vi "getPositionAllAxis.vi"(0 "connection ID":refnum<k5>, 5 "error":errorcluster) -> (14 "connection ID out":refnum<k5>, 15 "pos_nm_x":dbl, 16 "pos_nm_y":dbl, 17 "pos_nm_z":dbl, 19 "error out":errorcluster)   [LabVIEW 2016, in "amc_api.lvlib"]
doc: "This function returns the position of all three axes in nm\n If there is no positioner on one axis or the sensor is disabled, it returns -2147483648 nm instead"
uses:
  amc_api.lvlib
panel:
  out "jsonRespIn":string
  out "JSON-response":string="{\"jsonrpc\":\"2.0\",\"method\":\"\",\"params\":[5,1.245,true,\"name\"],\"id\":\"1\"}"
  out "JSON request":string
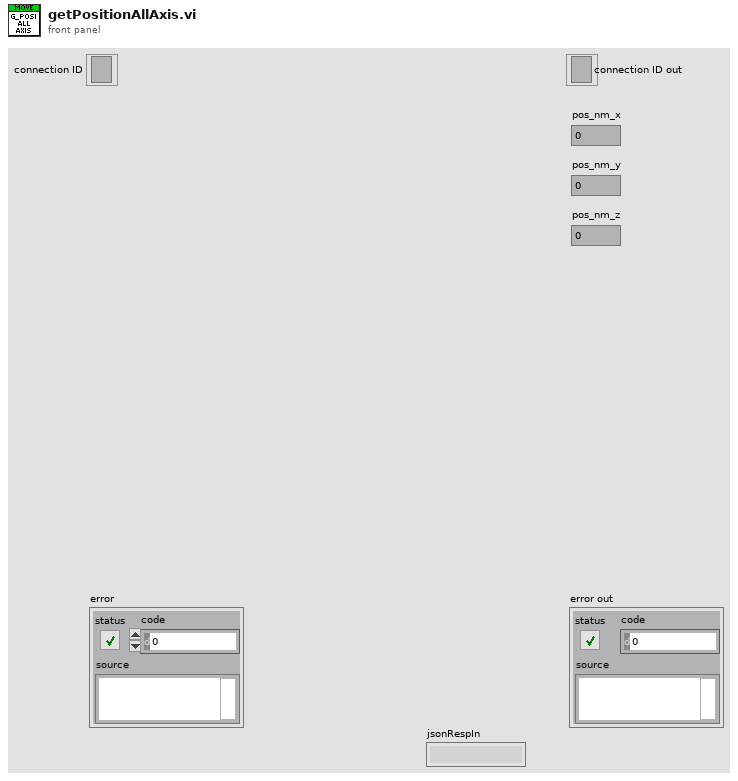
[diagram p1: front panel]
types:
  T1 = cluster{"jsonrpc":string, "method":string, "params":string[], "id":string, "api":i32, "pid":string}
  T2 = enum16{"Standard", "Buffered", "CRLF", "Immediate"}
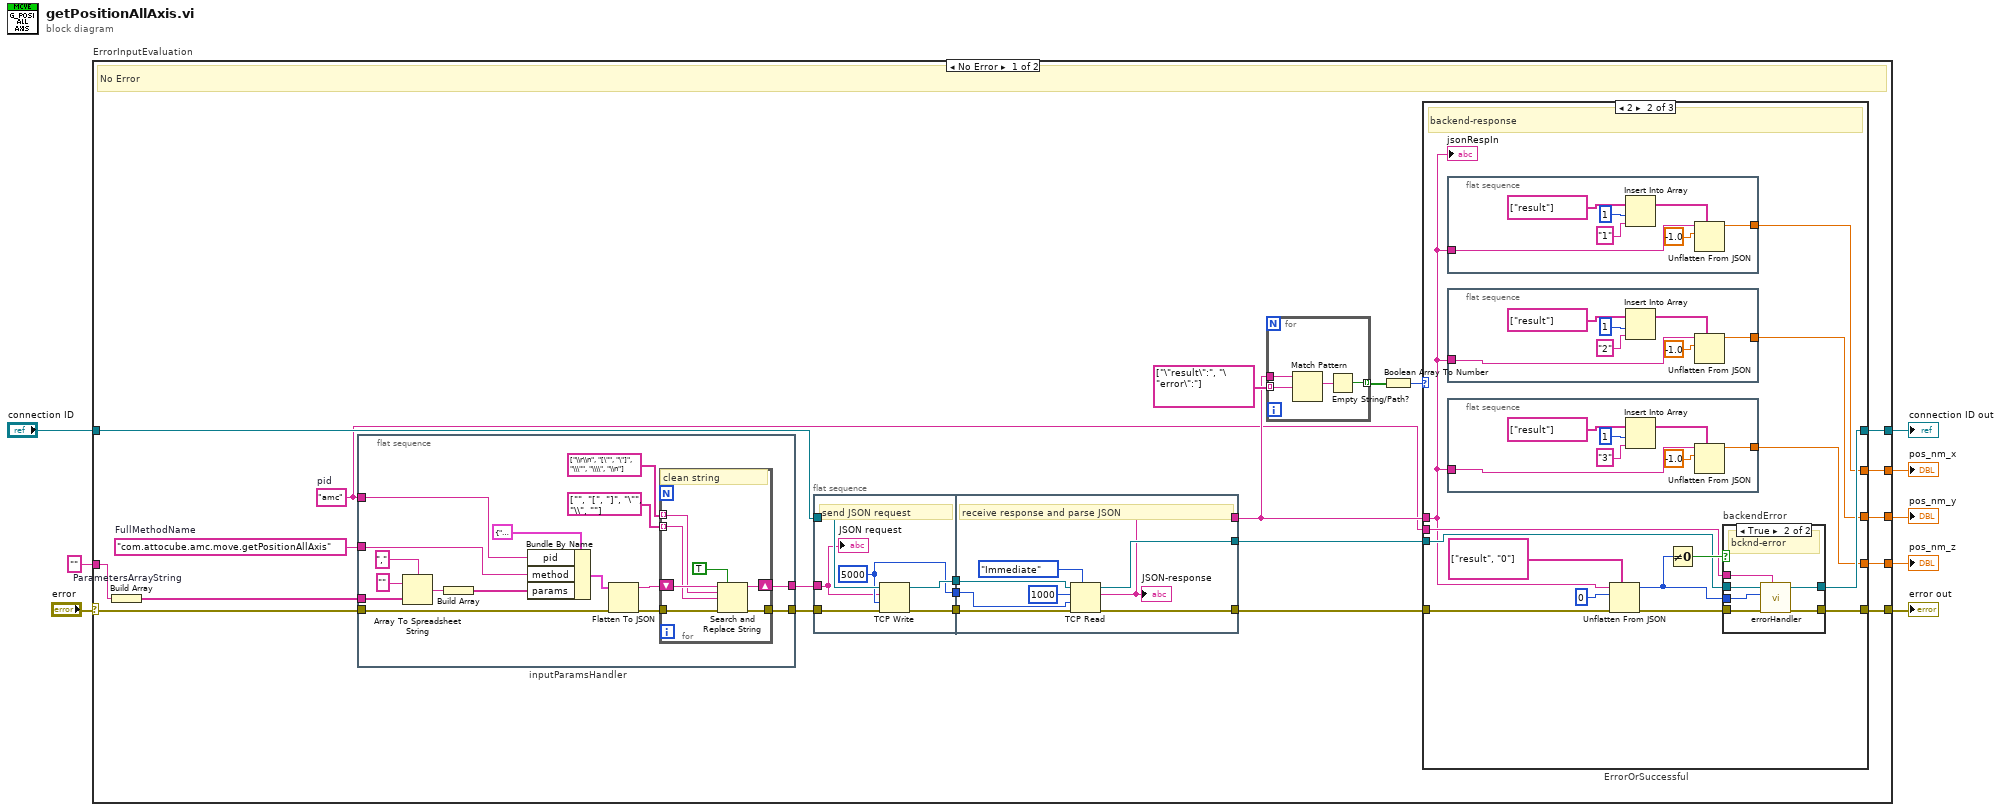
[diagram p0: block diagram]
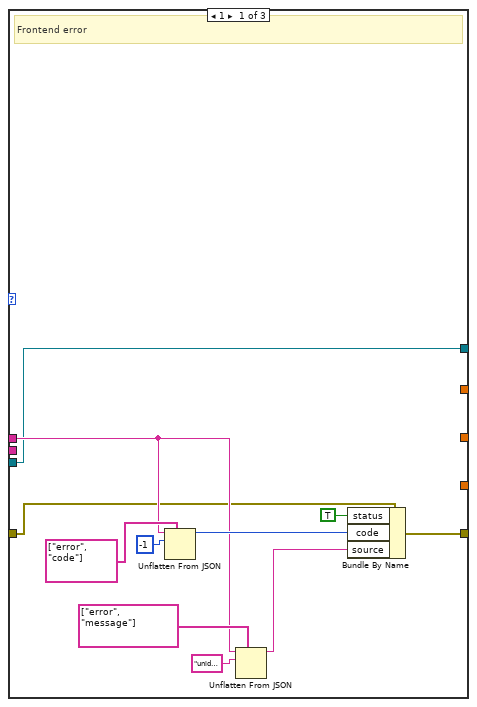
[diagram p2: hidden frame]
diagram:
  n1 = case "ErrorInputEvaluation" shown="No Error" "error" {
    selector: "error" -> [w23 w128]
    tunnel: "connection ID" -> [w27 w129]
    tunnel: [w14 w128] -> w7
    tunnel: [w15 w129] -> w6
    tunnel: "" -> [w12 _]
    tunnel: [w11 _] -> w3
    tunnel: [w10 _] -> w2
    tunnel: [w9 _] -> w1
    frame No Error {
      w13 = "amc"  # pid
      w24 = "com.attocube.amc.move.getPositionAllAxis"  # FullMethodName
      # "No Error"
      n2 = Build Array "ParametersArrayString"(w12) -> (w22:string[])
      n3 = flat-sequence "inputParamsHandler" {
        tunnel: [w92] -> w21
        tunnel: w22 -> [w98]
        tunnel: w23 -> [w97]
        tunnel: [w94] -> w20
        tunnel: w24 -> [w88]
        tunnel: w13 -> [w87]
        frame #0 {
          n4 = Array To Spreadsheet String(delimiter (Tab)=",", array=w98, 3:"" ("format string")) -> (spreadsheet string=w100:string)
          n5 = Build Array "Build Array"(w100) -> (w89:string[])
          n6 = Bundle By Name(cluster=T1 {"jsonrpc"="2.0", "method"="com.attocube.amc.res.setRESReadOutFreq", "params"=[], "id"="1", "api"=2, "pid"=""} ("Cluster"), "pid"=w87, "method"=w88, "params"=w89) -> (w99:T1)
          n7 = Flatten To JSON(anything=w99, error in (no error)=w97) -> (JSON string=w93:string, 11:w95:errorcluster)  [unwired: 1 in]
          n8 = for {
            tunnel: string[] ["\\r\\n", "[\"", "\"]", "\\\"", "\\\\", "\\n"] ("search string") -> [w106] mode=indexing
            tunnel: string[] ["", "[", "]", "\"", "\\", ""] ("replace string (\"\")") -> [w105] mode=indexing
            shift-right: [w108] -> w92
            shift-left: w93 -> [w107]
            tunnel: w95 -> [w104]
            tunnel: [w103] -> w94
            # "clean string"
            n9 = Search and Replace String(replace all?=TRUE ("replace all? (F)"), input string=w107, search string=w106, replace string=w105, error in=w104) -> (result string=w108:string, error out=w103:errorcluster)  [unwired: 3 in, 2 out]
          }
        }
      }
      n10 = flat-sequence {
        tunnel: w27 -> [w119]
        tunnel: [w117] -> w30
        tunnel: [w118] -> w29
        tunnel: w20 -> [w114]
        tunnel: [w116] -> w28
        tunnel: w21 -> [w115]
        tunnel: [w123] -> w19
        tunnel: w30 -> [w125]
        tunnel: w29 -> [w124]
        tunnel: [w121] -> w18
        tunnel: w28 -> [w122]
        tunnel: [w120] -> w17
        frame #0 {
          w116 = 5000 ("timeout ms (25000)")
          # "send JSON request"
          n11 = TCP Write(connection ID=w119, data in=w115, error in (no error)=w114, 9:w116) -> (connection ID out=w117:refnum<k5>, error out=w118:errorcluster)  [unwired: 1 out]
          "JSON request" <- w115
        }
        frame #1 {
          # "receive response and parse JSON"
          n12 = TCP Read(connection ID=w125, bytes to read=1000, error in (no error)=w124, 7:T2."Immediate" ("mode (standard)"), 9:w122) -> (connection ID out=w123:refnum<k5>, data out=w120:string, error out=w121:errorcluster)
          "JSON-response" <- w120
        }
      }
      n13 = for {
        tunnel: string[] ["\"result\":", "\"error\":"] ("path") -> [w112] mode=indexing
        tunnel: [w110] -> w25 mode=indexing
        tunnel: w17 -> [w113]
        n14 = Match Pattern(string=w113, regular expression=w112) -> (match substring=w111:string)  [unwired: 1 in, 3 out]
        n15 = Empty String/Path?(string/path=w111) -> (empty?=w110:bool)
      }
      n16 = Boolean Array To Number(Boolean array=w25) -> (number=w16:u32)
      n17 = case "ErrorOrSuccessful" shown="2" w16 {
        tunnel: w17 -> [w33 w47 _]
        tunnel: w19 -> [w31 w49 w86]
        tunnel: [w31 w48 w86] -> w15
        tunnel: [w34 w45 w85] -> w14
        tunnel: w18 -> [w32 w46 w85]
        tunnel: w13 -> [_ w50 _]
        tunnel: [_ w44 _] -> w11
        tunnel: [_ w43 _] -> w10
        tunnel: [_ w42 _] -> w9
        frame 1 {
          # "Frontend error"
          n18 = Unflatten From JSON(path=string[] ["error", "code"], JSON string=w33, type and defaults=-1) -> (value=w40:i32)  [unwired: 4 in, 1 out]
          n19 = Unflatten From JSON(path=string[] ["error", "message"], JSON string=w33, type and defaults="unidentified error") -> (value=w41:string)  [unwired: 4 in, 1 out]
          n20 = Bundle By Name(cluster=w32, "status"=TRUE, "code"=w40, "source"=w41) -> (w34:errorcluster)
        }
        frame 2 {
          # "backend-response"
          n21 = flat-sequence "out_double" {
            tunnel: [w70] -> w44
            tunnel: w47 -> [w72]
            frame #0 {
              n22 = Insert Into Array(array=string[] ["result"] ("path"), index=1, new element="1" ("idx")) -> (w74:string[])
              n23 = Unflatten From JSON(path=w74, JSON string=w72, type and defaults=-1.0 ("index")) -> (value=w70:dbl)  [unwired: 4 in, 1 out]
            }
          }
          n24 = flat-sequence "out_double" {
            tunnel: [w63] -> w43
            tunnel: w47 -> [w65]
            frame #0 {
              n25 = Insert Into Array(array=string[] ["result"] ("path"), index=1, new element="2" ("idx")) -> (w67:string[])
              n26 = Unflatten From JSON(path=w67, JSON string=w65, type and defaults=-1.0 ("index")) -> (value=w63:dbl)  [unwired: 4 in, 1 out]
            }
          }
          n27 = flat-sequence "out_double" {
            tunnel: [w56] -> w42
            tunnel: w47 -> [w58]
            frame #0 {
              n28 = Insert Into Array(array=string[] ["result"] ("path"), index=1, new element="3" ("idx")) -> (w60:string[])
              n29 = Unflatten From JSON(path=w60, JSON string=w58, type and defaults=-1.0 ("index")) -> (value=w56:dbl)  [unwired: 4 in, 1 out]
            }
          }
          n30 = Unflatten From JSON(path=string[] ["result", "0"], JSON string=w47, type and defaults=0, error in (no error)=w46) -> (value=w51:i32, error out=w53:errorcluster)  [unwired: 3 in]
          n31 = Not Equal To 0?(x=w51) -> (x != 0?=w52:bool)
          n32 = case "backendError" shown="True" w52 {
            tunnel: w51 -> [_ w84]
            tunnel: w53 -> [w78 w83]
            tunnel: [w77 w82] -> w48
            tunnel: [w78 w81] -> w45
            tunnel: w49 -> [w77 w80]
            tunnel: w50 -> [_ w79]
            frame False {
              # "successful"
            }
            frame True {
              # "bcknd-error"
              n33 = call "errorHandler.vi"("pid"=w79, "error in"=w83, "errNbr"=w84, "connection ID"=w80) -> ("error out 2"=w81:errorcluster, "connection ID out"=w82:refnum<k5>)  [unwired: 6 in]
            }
          }
          "jsonRespIn" <- w47
        }
        frame Default {
          # "NoResponse"
        }
      }
    }
    frame Error {
      # "Error"
    }
  }
  "error out" <- w7
  "connection ID out" <- w6
  "pos_nm_x" <- w3
  "pos_nm_y" <- w2
  "pos_nm_z" <- w1
